vi "Write Selected Tests.vi"(8 "error in (no error)":errorcluster, 10 "Selected Tests":bool[](array[boolean]), 11 "Test Selector in":refnum<class "Test Selector.lvclass">) -> (0 "error out":errorcluster, 3 "Test Selector out":refnum<class "Test Selector.lvclass">)   [LabVIEW 2019, in "Test Selector.lvlib" / "Test Selector.lvclass"]
uses:
  Test Selector.lvclass
  Test Selector.lvclass/Test Selector.ctl
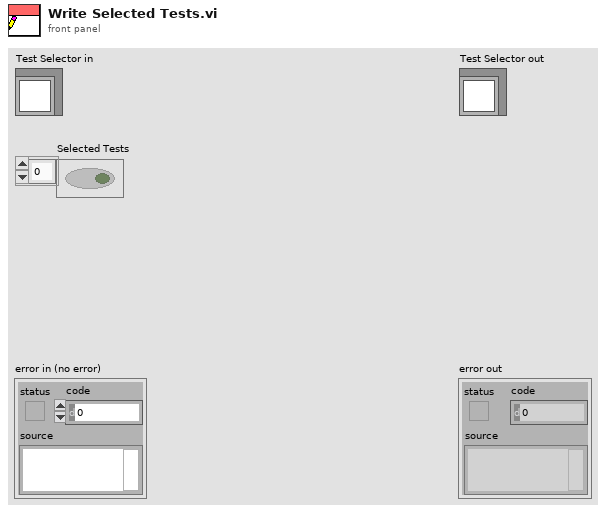
[diagram p1: front panel]
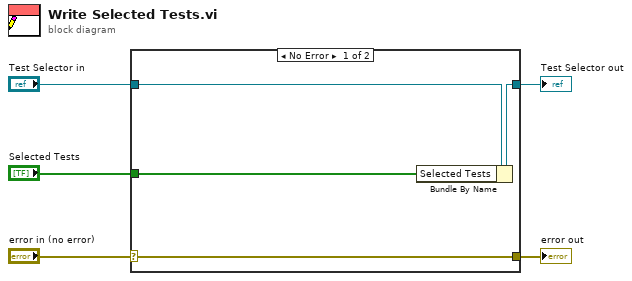
[diagram p0: block diagram]
diagram:
  n1 = case shown="No Error" "error in (no error)" {
    selector: "error in (no error)" -> [w9 w10]
    tunnel: [w9 w10] -> w4
    tunnel: [w7 w11] -> w2
    tunnel: "Test Selector in" -> [w8 w11]
    tunnel: "Selected Tests" -> [w6 _]
    frame No Error {
      n2 = Bundle By Name(cluster=w8, "Selected Tests"=w6) -> (w7:refnum<class "Test Selector.lvclass">)
    }
    frame Error {
    }
  }
  "error out" <- w4
  "Test Selector out" <- w2
